vi "Thread Loop.vi"(8 "error in (no error)":errorcluster, 11 "Entry Console in":refnum<class "Entry Console.lvclass">) -> (0 "error out":errorcluster, 3 "Entry Console out":refnum<class "Entry Console.lvclass">)   [LabVIEW 2019, in "Entry Console.lvlib" / "Entry Console.lvclass"]
uses:
  Entry Console.lvclass
  Thread/Thread.lvclass
  Queue/Queue.lvclass
  Entry Console Start Msg/Register Entry Console References.lvclass
  C:/Users/nitest/Downloads/Sample Exams/Carwash (100529-01)/Actor Objects/Message/Message.lvclass
  Wash Step Selection.ctl
panel:
  in  "Wash Step Selection Buttons":T1={"Blank Button"=FALSE, "Blank Button 2"=FALSE, "Blank Button 3"=FALSE, "Blank Button 4"=TRUE, "Blank Button 5"=FALSE, "Blank Button 6"=FALSE, "Blank Button 7"=FALSE, "Blank Button 8"=FALSE}
  in  "Start Wash":bool
  # "[Covers: UI2]"
  # "[Covers: UI2A]"
  # "[Covers: UI2A1]"
  # "[Covers: UI2B]"
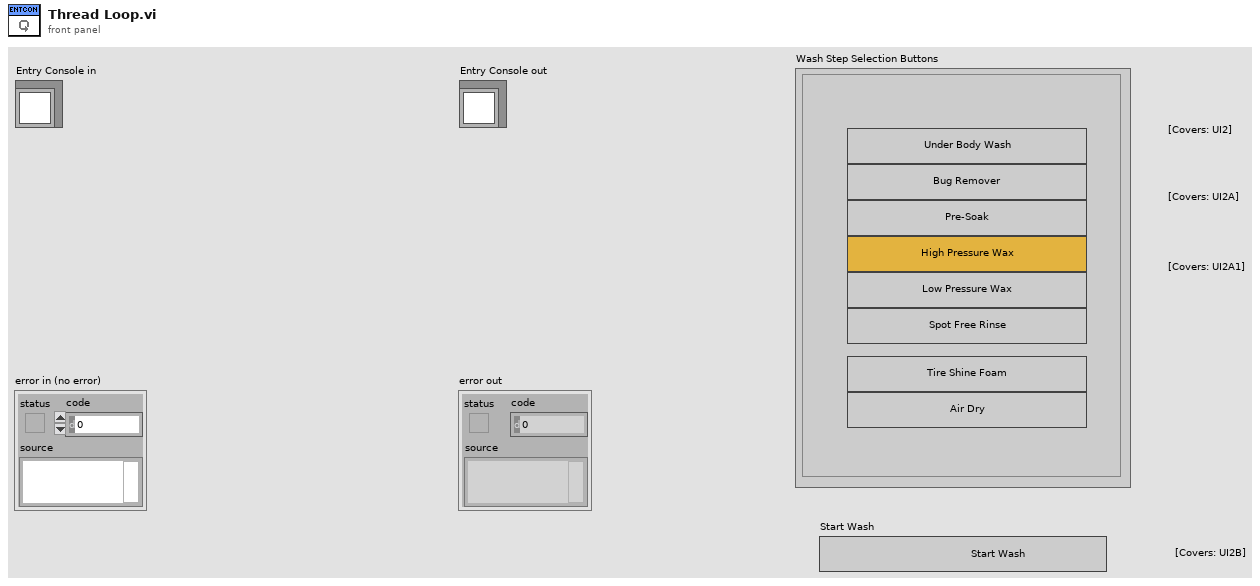
[diagram p1: front panel]
types:
  T1 = typedef "Entry Console.lvlib/Entry Console.lvclass/Wash Step Selection.ctl" = cluster{"Blank Button":bool, "Blank Button 2":bool, "Blank Button 3":bool, "Blank Button 4":bool, "Blank Button 5":bool, "Blank Button 6":bool, "Blank Button 7":bool, "Blank Button 8":bool}
  T2 = enum32{"Invalid", "Standard", "Closed", "Hidden", "Minimized", "Maximized"}
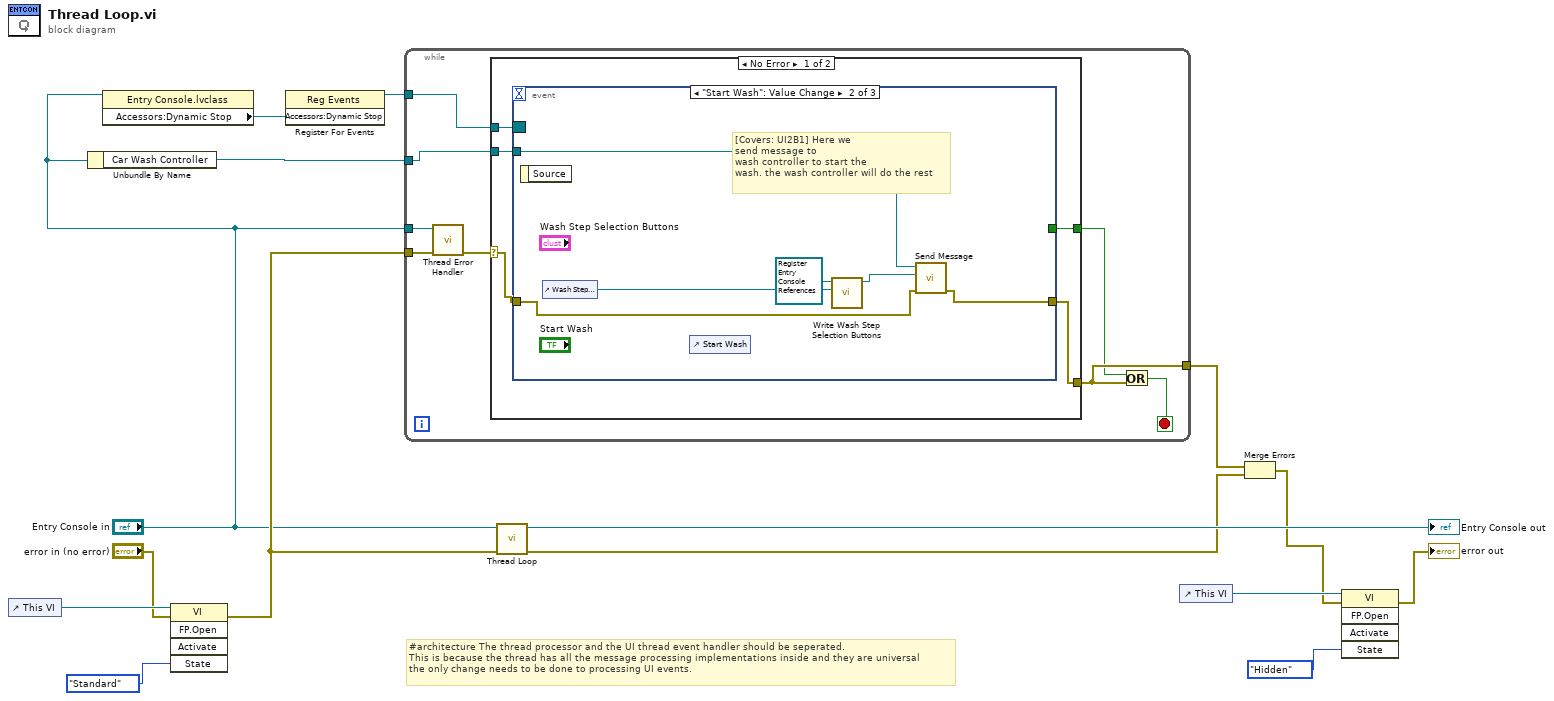
[diagram p0: block diagram]
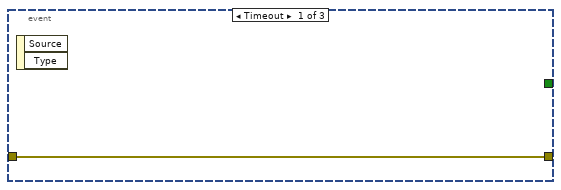
[diagram p2: hidden frame]
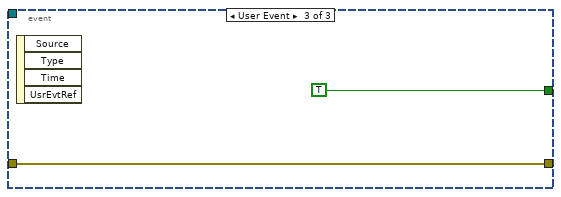
[diagram p3: hidden frame]
diagram:
  # "#architecture The thread processor and the UI thread event handler should be seperated.\nThis is because the thread has all the message processing implementations inside and they are universal\nthe only change needs to be done to processing UI events."
  n1 = control-ref of="This VI"() -> (w11:refnum<vi>)
  n2 = Unbundle By Name("Entry Console in") -> ("Car Wash Controller"=w14:refnum<class "Queue.lvclass">)
  n3 = property class="Entry Console.lvclass"(reference="Entry Console in") -> ("Accessors:Dynamic Stop"=w2:refnum<user-event>)  [unwired: 1 in, 2 out]
  n4 = invoke class="VI" method="FP.Open"(reference=w11, error in="error in (no error)", "State"=T2."Standard") -> (error out=w8:errorcluster)  [unwired: 2 in, 4 out]
  n5 = register-events(w2) -> (reference out=w1:refnum<event-registration>)  [unwired: 2 in, 1 out]
  n6 = while {
    tunnel: w8 -> [w23]
    tunnel: "Entry Console in" -> [w22]
    tunnel: w14 -> [w19]
    tunnel: [w18] -> w12
    tunnel: w1 -> [w17]
    stop <- w20 stop-if-true
    n7 = call-dynamic "Thread Error Handler.vi"("error in (no error)"=w23, "Thread in"=w22) -> ("error out"=w21:errorcluster)  [unwired: 8 in, 1 out]
    n8 = case shown="No Error" w21 {
      selector: w21 -> [w24 w38]
      tunnel: [w25 w38] -> w18
      tunnel: w19 -> [w28 _]
      tunnel: w17 -> [w27 _]
      tunnel: [w26 _] -> w16
      frame No Error {
        n9 = event shown="[1] \"Start Wash\": Value Change" {
          selector: w27 -> [_ _ _]
          dyn-events: _ -> [_ _ _]
          timeout: _ -> [_ _ _]
          tunnel: w28 -> [_ w35 _]
          tunnel: [_ _ TRUE] -> w26
          tunnel: [w29 w30 w36] -> w25
          tunnel: w24 -> [w29 w31 w36]
          event Timeout {
            n10 = event-data() -> ()  [unwired: 1 in, 2 out]
          }
          event "Start Wash": Value Change {
            # "[Covers: UI2B1] Here we\nsend message to \nwash controller to start the\nwash. the wash controller will do the rest"
            n11 = event-data() -> ()  [unwired: 1 in, 1 out]
            n12 = control-ref of="Wash Step Selection Buttons"() -> (w34:refnum<vi>)
            n13 = control-ref of="Start Wash"() -> ()  [unwired: 1 out]
            n14 = call "Write Wash Step Selection Buttons.vi"("Wash Step Selection Buttons"=w34, "Entry Console Start Msg in"=refnum<class "Register Entry Console References.lvclass"> refnum) -> ("Entry Console Start Msg out"=w32:refnum<class "Register Entry Console References.lvclass">)  [unwired: 9 in]
            n15 = call "Send Message.vi"("error in (no error)"=w31, "Architecture.lvlib:Message.lvclass"=w32, "Queue in"=w35) -> ("error out"=w30:errorcluster)  [unwired: 7 in, 1 out]
          }
          event User Event {
            n16 = event-data() -> ()  [unwired: 1 in, 4 out]
          }
        }
      }
      frame Error {
      }
    }
    n17 = Or(x=w16, y=w18) -> (x .or. y?=w20:bool)
  }
  n18 = call-parent "Thread Loop.vi"("error in (no error)"=w8, "Thread in"="Entry Console in") -> ("error out"=w13:errorcluster, "Thread out"=→"Entry Console out":refnum<class "Entry Console.lvclass">)  [unwired: 8 in]
  n19 = control-ref of="This VI"() -> (w7:refnum<vi>)
  n20 = Merge Errors(w12, w13) -> (w5:errorcluster)
  n21 = invoke class="VI" method="FP.Open"(reference=w7, error in=w5, "State"=T2."Hidden") -> (error out=→"error out":errorcluster)  [unwired: 2 in, 4 out]
